vi "SetNumbersAndOperationMethod Wrapper - Reentrant.vi"(6 "error in (no error)":errorcluster, 8 "Operator":enum16{"Add", "Divide", "Multiple", "Subtract"}(ring), 9 "Numeric 2":dbl, 10 "Numeric":dbl, 11 "SimpleArithmetic in":refnum<class "SimpleArithmetic - Reentrant.lvclass">) -> (0 "error out":errorcluster, 3 "SimpleArithmetic out":refnum<class "SimpleArithmetic - Reentrant.lvclass">)   [LabVIEW 2010]
uses:
  SimpleArithmetic - Reentrant.lvclass
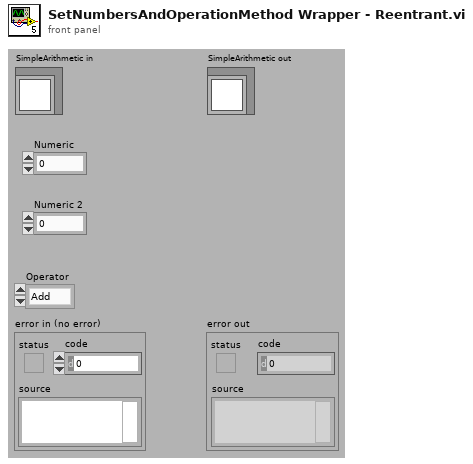
[diagram p1: front panel]
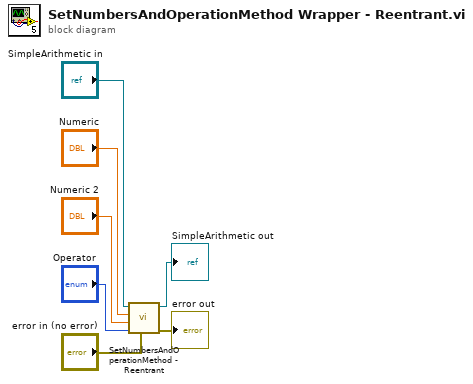
[diagram p0: block diagram]
diagram:
  n1 = call "SetNumbersAndOperationMethod - Reentrant.vi"("error in (no error)"="error in (no error)", "Operator"="Operator", "Numeric 2"="Numeric 2", "Numeric"="Numeric", "SimpleArithmetic in"="SimpleArithmetic in") -> ("error out"=→"error out":errorcluster, "SimpleArithmetic out"=→"SimpleArithmetic out":refnum<class "SimpleArithmetic - Reentrant.lvclass">)  [unwired: 5 in]
